vi "CleanUp.vi"(0 "object in":refnum<class "Battleship.lvclass">, 5 "error in (no error)":errorcluster) -> (14 "object out":refnum<class "Battleship.lvclass">, 19 "error out":errorcluster)   [LabVIEW 2015, in "Battleship.lvclass"]
doc: "Cleans up all resources used by this class."
uses:
  Battleship.lvclass
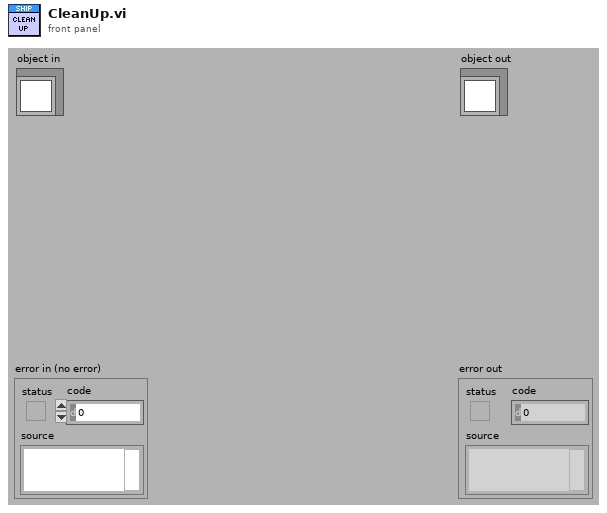
[diagram p1: front panel]
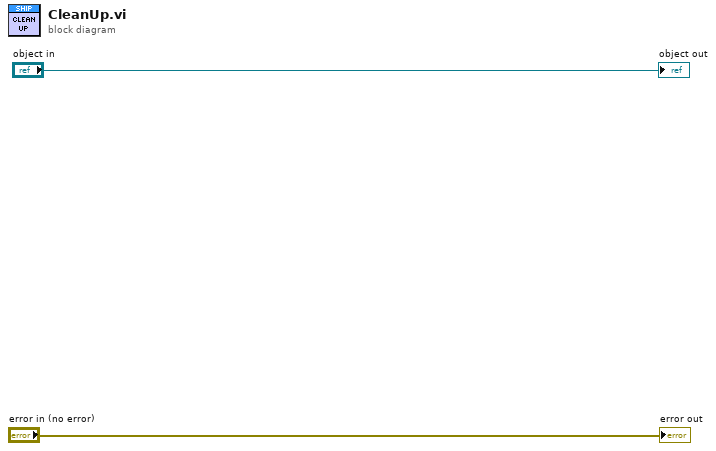
[diagram p0: block diagram]
diagram:
  "error out" <- "error in (no error)"
  "object out" <- "object in"
